vi "Get DDS Sweep Start Freq.vi"(11 "channel_index":u8) -> (3 "function return":dbl)   [LabVIEW 2021, in "vmmso.lvlib"]
doc: "DLL_API double WINAPI GetDDSSweepStartFreq(unsigned char channel_index);"
uses:
  vmmso.lvlib
  vmmso.dll
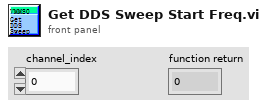
[diagram p1: front panel]
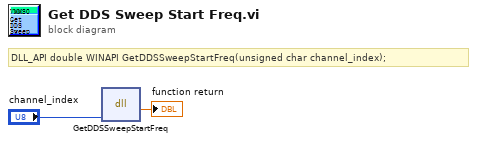
[diagram p0: block diagram]
diagram:
  # "DLL_API double WINAPI GetDDSSweepStartFreq(unsigned char channel_index);"
  n1 = dll-call lib="D:/labviewdemo/LabviewDemo 21/vmmso/vmmso.*" fn="GetDDSSweepStartFreq"("channel_index"="channel_index") -> (→"function return":dbl)  [unwired: 4 in, 2 out]
